vi "red.vi"() -> (3 "red 5":i32)   [LabVIEW 2019]
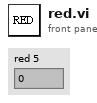
[diagram p1: front panel]
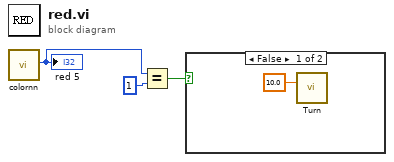
[diagram p0: block diagram]
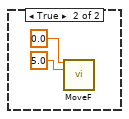
[diagram p2: hidden frame]
diagram:
  n1 = call "colornn.vi"() -> ("red"=w1:i32)  [unwired: 14 in, 5 out]
  "red 5" <- w1
  n2 = Equal?(x=w1, y=1) -> (x = y?=w3:bool)
  n3 = case shown="False" w3 {
    frame False {
      n4 = call "Turn.vi"("¨¤«×"=10.0) -> ()  [unwired: 14 in, 1 out]
    }
    frame True {
      n5 = call "MoveF.vi"("X"=0.0, "Y"=5.0) -> ()  [unwired: 13 in, 1 out]
    }
  }
